vi "Handle setConfiguration.vi"(8 "error in (no error)":errorcluster, 10 "setConfiguration":variant, 11 "Inst.Xeryon-Rotator in":refnum<class "Inst.Xeryon-Rotator.lvclass">) -> (0 "error out":errorcluster, 3 "Inst.Xeryon-Rotator out":refnum<class "Inst.Xeryon-Rotator.lvclass">)   [LabVIEW 2019, in "Inst.Xeryon-Rotator.lvclass"]
uses:
  Inst.Xeryon-Rotator.lvclass
  45e4b271-6884-462c-ad3a-d505ab08eb62.vi
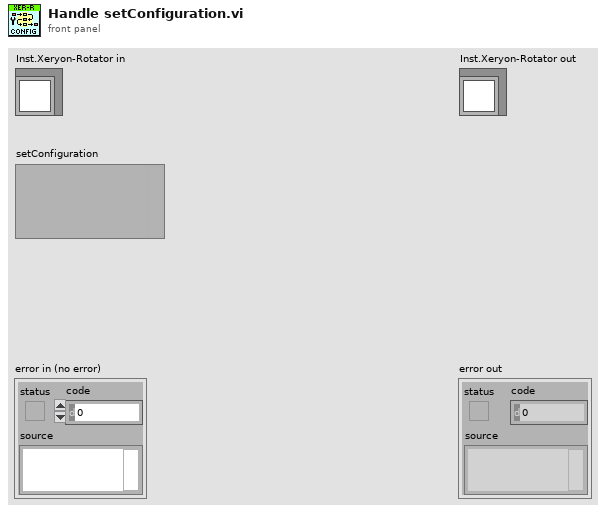
[diagram p1: front panel]
types:
  T1 = typedef "Inst.Xeryon-Rotator.lvclass/Inst.Xeryon-Rotator.Configuration--Cluster.ctl" = cluster{"Example Setting 1":dbl, "Example Setting 2":dbl, "Example Setting 3":string}
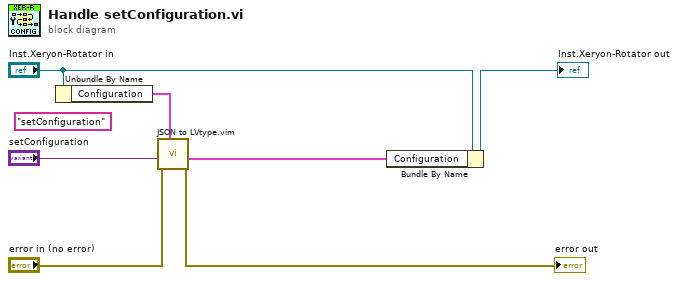
[diagram p0: block diagram]
diagram:
  (unwired) "setConfiguration" ("Command")
  n1 = Unbundle By Name("Inst.Xeryon-Rotator in") -> ("Configuration"=w6:T1)
  n2 = call "JSON to LVtype.vim"("type"=w6, "error in (no error)"="error in (no error)", "JSON Data in"="setConfiguration") -> ("error out"=→"error out":errorcluster, "Data out"=w1:T1)  [unwired: 7 in]
  n3 = Bundle By Name(cluster="Inst.Xeryon-Rotator in", "Configuration"=w1) -> (→"Inst.Xeryon-Rotator out":refnum<class "Inst.Xeryon-Rotator.lvclass">)
